vi "Get Entries.vi"(8 "error in (no error)":errorcluster, 11 "Results in":refnum<class "Results.lvclass">) -> (0 "error out":errorcluster, 2 "Entries":T1[](array[typedef]), 3 "Results out":refnum<class "Results.lvclass">)   [LabVIEW 2020, in "Tester.lvlib" / "Results.lvclass"]
uses:
  Results.lvclass
  Entry.ctl
  Result.ctl
  Results.lvclass/Results.ctl
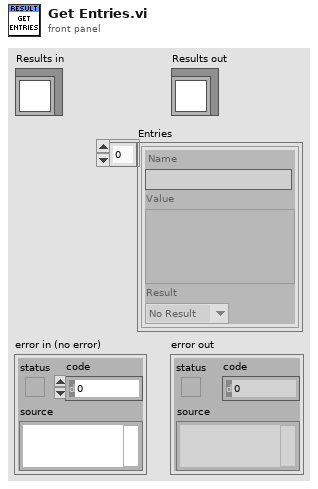
[diagram p1: front panel]
types:
  T1 = typedef "Tester.lvlib/Results.lvclass/Entry.ctl" = cluster{"Name":string, "Value":variant, "Result":T2}
  T2 = typedef "Tester.lvlib/Results.lvclass/Result.ctl" = enum16{"No Result", "Pass", "Fail", "Error", "Abort"}
  T3 = typedef "Tester.lvlib/Results.lvclass/Results Ref.ctl" = cluster{"Entries":T1[], "Overall Result":T2}
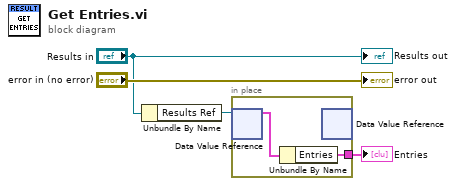
[diagram p0: block diagram]
diagram:
  n1 = Unbundle By Name("Results in") -> ("Results Ref"=w3:refnum<data-value>)
  n2 = in-place {
    in-place-border: [w5] -> w1
    n3 = in-place-dvr #1(w3) -> (w6:T3)  [unwired: 1 out]
    n4 = Unbundle By Name(w6) -> ("Entries"=w5:T1[])
    n5 = in-place-dvr #1() -> ()  [unwired: 1 in, 2 out]
  }
  "Entries" <- w1
  "error out" <- "error in (no error)"
  "Results out" <- "Results in"
